vi "writeToXML.vi"(8 "error in (no error)":errorcluster, 10 "ClassLabel":string, 11 "MccEnable in":refnum<class "MccEnable.lvclass">) -> (0 "error out":errorcluster, 2 "XML out":string, 3 "MccEnable out":refnum<class "MccEnable.lvclass">)   [LabVIEW 2022 SP3, in "TCSDataDefinitions.lvlib" / "TCSMountControlCommand.lvlib" / "CommandsForAllAxes.lvlib" / "MccEnable.lvclass"]
uses:
  MccEnable.lvclass
  CommandsForAllAxes.lvclass
  <userlib>/Common/XML/XMLGenerator/XMLGenerator.lvclass
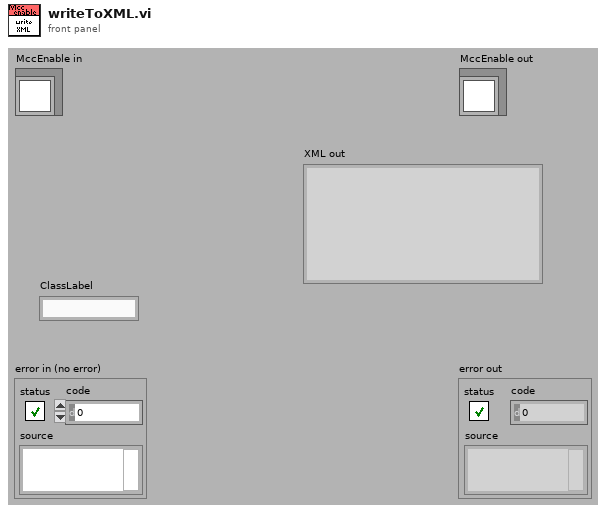
[diagram p1: front panel]
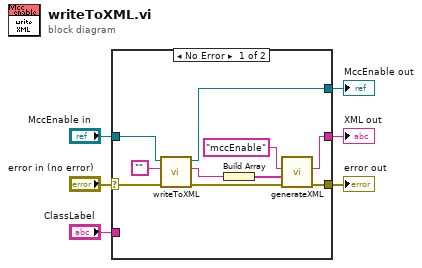
[diagram p0: block diagram]
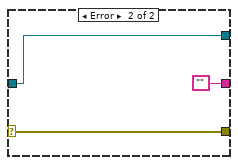
[diagram p2: hidden frame]
diagram:
  n1 = case shown="No Error" "error in (no error)" {
    selector: "error in (no error)" -> [w8 w19]
    tunnel: [w7 w19] -> w5
    tunnel: [w13 w18] -> w3
    tunnel: "MccEnable in" -> [w14 w18]
    tunnel: [w10 ""] -> w2
    tunnel: "ClassLabel" -> [_ _]
    frame No Error {
      n2 = call-parent "writeToXML.vi"("error in (no error)"=w8, "ClassLabel"="", "CommandsForAllAxes in"=w14) -> ("error out"=w9:errorcluster, "XMLout"=w15:string, "CommandsForAllAxes out"=w13:refnum<class "MccEnable.lvclass">)  [unwired: 6 in]
      n3 = Build Array(w15) -> (w12:string[])
      n4 = call <userlib>:"generateXML.vi"("error in"=w9, "childrenXML"=w12, "elementName"="mccEnable" ("Class Label")) -> ("error out"=w7:errorcluster, "XML out"=w10:string)  [unwired: 6 in, 1 out]
    }
    frame Error {
    }
  }
  "error out" <- w5
  "MccEnable out" <- w3
  "XML out" <- w2
